vi "Global_ACT_Data Out.vi"() -> ()   [LabVIEW 2023, in "Intake_ACT.lvlib"]
uses:
  startup.rtexe/Intake_ACT.lvlib
  Cluster_Shooter Status.ctl
  startup.rtexe/Cluster_Speed Sensor Values.ctl
  startup.rtexe/Cluster_Velocity Values.ctl
  startup.rtexe/Cluster_Voltage Values.ctl
  startup.rtexe/CTRE_Phoenix_MotorControl_ControlMode.ctl
  startup.rtexe/Shooter_ACT.lvlib
panel:
  in  "ACT_Intake_Control Mode":T1 items=["PercentOutput"=0, "Position"=1, "Velocity"=2, "Current"=3, "Follower"=5, "MotionProfile"=6, "MotionMagic"=7, "MotionProfileArc"=10, "Disabled"=15]
  in  "ACT_Intake_Status":T2
  in  "ACT_Intake Motor Value":dbl
  in  "ACT_Intake_CycleTime(S)":dbl
  # "The Names of the Data items in the Global Variable MUST describe who the Single Writer is\nFor Actuator Globals the the naming convention is\n   \nACT_Lib Name_Data Name\n\nExamples:\nACT_Drive_X axis\nACT_Hopper_AgitatorSpeed"
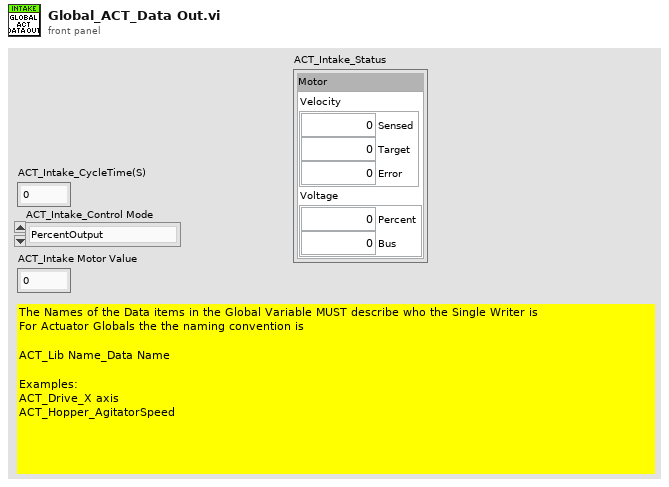
[diagram p1: front panel]
types:
  T1 = typedef "CTRE_Phoenix_MotorControl_ControlMode.ctl" = u16
  T2 = typedef "Intake_ACT.lvlib/Cluster_Shooter Status.ctl" = cluster{"Motor":T3}
  T3 = typedef "Cluster_Speed Sensor Values.ctl" = cluster{"Velocity":T4, "Voltage":T5}
  T4 = typedef "Shooter_ACT.lvlib/Cluster_Velocity Values.ctl" = cluster{"Sensed":dbl, "Target":dbl, "Error":dbl}
  T5 = typedef "Shooter_ACT.lvlib/Cluster_Voltage Values.ctl" = cluster{"Percent":dbl, "Bus":dbl}
diagram:
